vi "capstone2 ver 2.vi"() -> ()   [LabVIEW 2016]
uses:
  <instrlib>/Dynamixel Motor/Public/Motor Operation/Low Level/Baud Setting.ctl
  <vilib>/myRIO/Instrument Drivers/Onboard IO/DIO/typedefs/DIO Reference.ctl
  <vilib>/myRIO/Common/Instrument Driver Framework/Utilities/typedefs/myRIO Generic Hardware Reference.ctl
  <vilib>/myRIO/Common/Instrument Driver Framework/Utilities/typedefs/Hardware Version Enum.ctl
  <vilib>/myRIO/Common/Instrument Driver Framework/Utilities/typedefs/myRIO v1.0 Reference.ctl
  <vilib>/myRIO/Common/Instrument Driver Framework/Utilities/typedefs/Generic FPGA Reference.ctl
  <vilib>/myRIO/Common/Instrument Driver Framework/myRIO v1.0/DIO/typedefs/DIO Channels List.ctl
  <vilib>/myRIO/Common/Instrument Driver Framework/myRIO v1.0/DIO/typedefs/DIO Channels Enum.ctl
  <vilib>/userdefined/High Color/nirio_resource_hc.ctl
  <vilib>/myRIO/Common/Instrument Driver Framework/Utilities/vis/Is FPGA Ref Available.vi
  <vilib>/myRIO/Common/Instrument Driver Framework/myRIO v1.0/DIO/vis/myRIO v1.1 Open DIO.vi
  <vilib>/myRIO/Instrument Drivers/Onboard IO/DIO/vis/Write.vi
  <vilib>/myRIO/Common/Instrument Driver Framework/Utilities/vis/Validate Channels.vi
  <vilib>/myRIO/Common/Instrument Driver Framework/myRIO v1.0/DIO/vis/myRIO v1.0 Reserve DIO.vi
  <vilib>/myRIO/Common/Instrument Driver Framework/myRIO v1.0/UART/vis/myRIO v1.0 Close UART.vi
  <vilib>/myRIO/Common/Instrument Driver Framework/myRIO v1.0/Resource Manager/vis/myRIO v1.0 Reserve Channel List.vi
  <vilib>/myRIO/Common/Instrument Driver Framework/myRIO v1.0/DIO/vis/myRIO v1.0 Build MUX Configuration DIO.vi
  <vilib>/myRIO/Common/Instrument Driver Framework/myRIO v1.0/Resource Manager/vis/myRIO v1.0 Reserve Channel.vi
  <vilib>/myRIO/Common/Instrument Driver Framework/myRIO v1.0/Resource Manager/vis/myRIO v1.0 Unreserve Channel.vi
  <vilib>/myRIO/Common/Instrument Driver Framework/myRIO v1.0/Resource Manager/vis/myRIO v1.0 Create Configuration List.vi
  <vilib>/myRIO/Common/Instrument Driver Framework/myRIO v1.0/Resource Manager/vis/myRIO v1.0 Build Mutex Name.vi
  <vilib>/Utility/VariantDataType/GetNumericInfo.vi
  <vilib>/Utility/error.llb/Error Cluster From Error Code.vi
  <vilib>/myRIO/Common/Instrument Driver Framework/myRIO v1.0/myRIO v1.1 Open.vi
  <vilib>/myRIO/Common/Instrument Driver Framework/Utilities/vis/IO Manager.vi
  <vilib>/myRIO/Common/Instrument Driver Framework/Utilities/vis/Configuration Manager.vi
  <vilib>/myRIO/Common/Instrument Driver Framework/myRIO v1.0/Resource Manager/vis/myRIO v1.0 Configure IO.vi
  <vilib>/myRIO/Common/Instrument Driver Framework/myRIO v1.0/myRIO v1.0 Close.vi
  <vilib>/myRIO/Common/Instrument Driver Framework/myRIO v1.0/DIO/vis/myRIO v1.0 Write DIO.vi
  <vilib>/myRIO/Common/Instrument Driver Framework/Utilities/vis/FPGA Ref Manager.vi
  <vilib>/myRIO/Common/Instrument Driver Framework/myRIO v1.0/myRIO v1.0 Reset FPGA.vi
  <vilib>/myRIO/Common/Instrument Driver Framework/myRIO v1.0/IRQ/vis/myRIO v1.0 IRQ Info FGV.vi
  <vilib>/myRIO/Common/Instrument Driver Framework/myRIO v1.0/IRQ/vis/myRIO v1.0 Timer IRQ Info FGV.vi
  <vilib>/myRIO/Common/Instrument Driver Framework/myRIO v1.0/IRQ/vis/myRIO v1.0 ISR Agent.vi
  <vilib>/myRIO/Express VI/Onboard Devices/LED/LED Express VI.xnode
  <vilib>/myRIO/Instrument Drivers/Onboard IO/DIO/vis/myRIO DIO Open.xnode
  <instrlib>/Dynamixel Motor/Dynamixel Motor.lvlib
  <vilib>/myRIO/Instrument Drivers/Onboard IO/DIO/DIO.lvlib
  <vilib>/myRIO/Instrument Drivers/Utilities/Utilities.lvlib
panel:
  in  "main stop":bool
  out "RT TCP Loop time":u32
  out "motor temp":cluster{"0":sgl, "1":sgl, "2":sgl, "3":sgl}
  out "value":T1
  out "TCP Read data":string
  in  "정지":bool
  out "error out":errorcluster
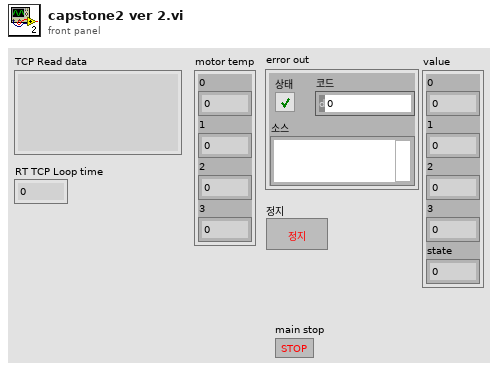
[diagram p1: front panel]
types:
  T1 = cluster{"0":sgl, "1":sgl, "2":sgl, "3":sgl, "state":sgl}
  T2 = typedef "DIO.lvlib/DIO Reference.ctl" = cluster{"myRIO Reference":T3, "DIO Channels List":T7}
  T3 = typedef "myRIO Generic Hardware Reference.ctl" = cluster{"myRIO Model":T4, "myRIO Hardware Reference":T5}
  T4 = typedef "Hardware Version Enum.ctl" = enum16{"Unknown", "myRIO-1900", "myRIO-1950", "roboRIO", "NI ELVIS RIO CM"}
  T5 = typedef "myRIO v1.0 Reference.ctl" = cluster{"Generic FPGA Reference":T6, "Allow multiple opens":bool}
  T6 = typedef "Generic FPGA Reference.ctl" = refnum<k20>
  T7 = typedef "DIO Channels List.ctl" = T8[]
  T8 = typedef "DIO Channels Enum.ctl" = enum16{"Not Connected", "C/DIO0", "C/DIO1", "C/DIO2", "C/DIO3", "C/DIO4", "C/DIO5", "C/DIO6", "C/DIO7", "A/DIO0", "A/DIO1", "A/DIO2", "A/DIO3", "A/DIO4", "A/DIO5", "A/DIO6", "A/DIO7", "A/DIO8", "A/DIO9", "A/DIO10", "A/DIO11", "A/DIO12", "A/DIO13", "A/DIO14", "A/DIO15", "B/DIO0", "B/DIO1", "B/DIO2", "B/DIO3", "B/DIO4", "B/DIO5", "B/DIO6", "B/DIO7", "B/DIO8", "B/DIO9", "B/DIO10", "B/DIO11", "B/DIO12", "B/DIO13", "B/DIO14", "B/DIO15", "LED0", "LED1", "LED2", "LED3", "Button0", "DIO/DIO0", "DIO/DIO1", "DIO/DIO2", "DIO/DIO3", "DIO/DIO4", "DIO/DIO5", "DIO/DIO6", "DIO/DIO7", "DIO/DIO8", "DIO/DIO9", "SPI/CS0", "SPI/CS1", "SPI/CS2", "SPI/CS3", "LED RADIO (Green)", "LED RADIO (Red)", "LED COMM (Green)", "LED COMM (Red)", "LED MODE (Green)", "LED MODE (Red)"}
  T9 = typedef "nirio_resource_hc.ctl" = tag
  T10 = cluster{"0":sgl, "1":sgl, "2":sgl, "3":sgl, "state":i32}
  T11 = typedef "Dynamixel Motor.lvlib/Baud Setting.ctl" = u8
  T12 = enum16{"big-endian, network order", "native, host order", "little-endian"}
  T13 = cluster{"Temperature (C)":u8, "Temperature (C)":u8, "Temperature (C)":u8, "Temperature (C)":u8}
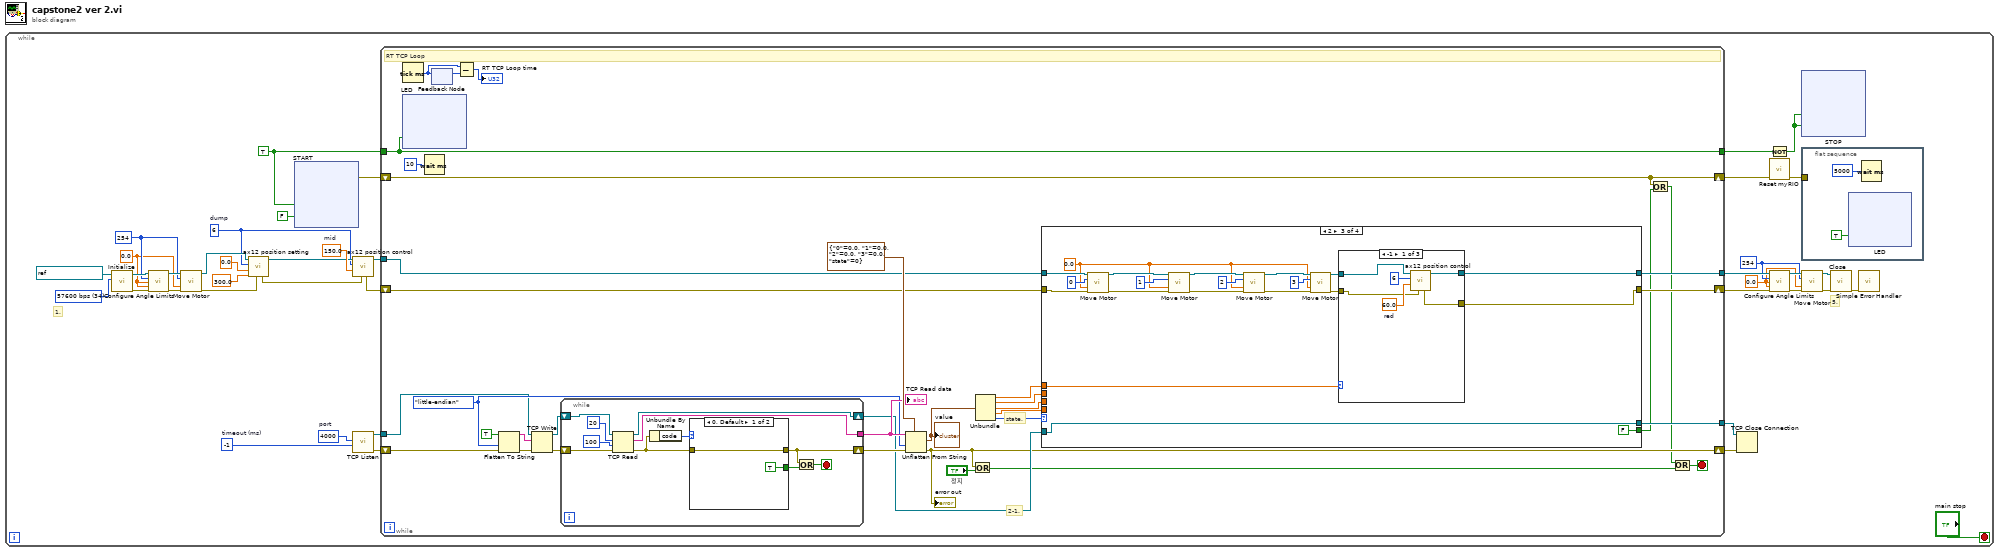
[diagram p0: block diagram]
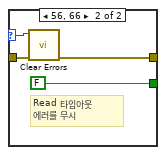
[diagram p2: hidden frame]
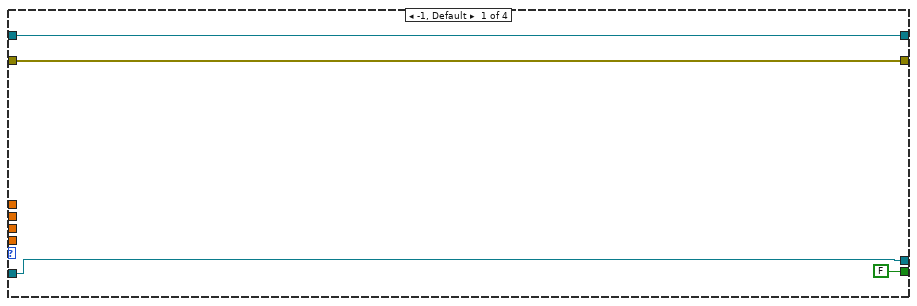
[diagram p3: hidden frame]
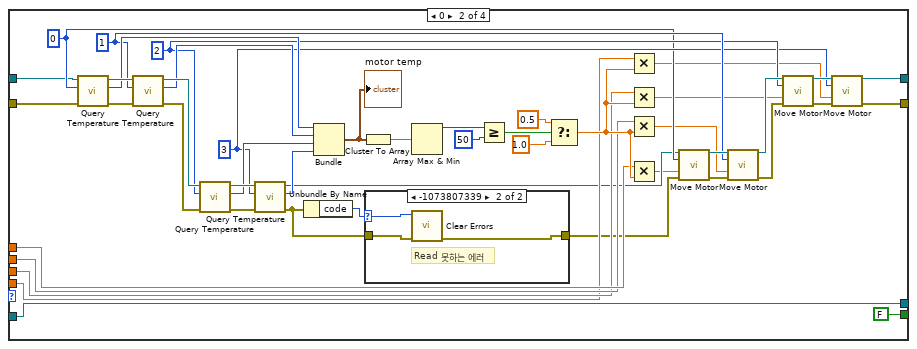
[diagram p4: hidden frame]
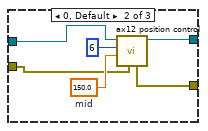
[diagram p6: hidden frame]
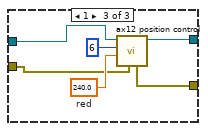
[diagram p7: hidden frame]
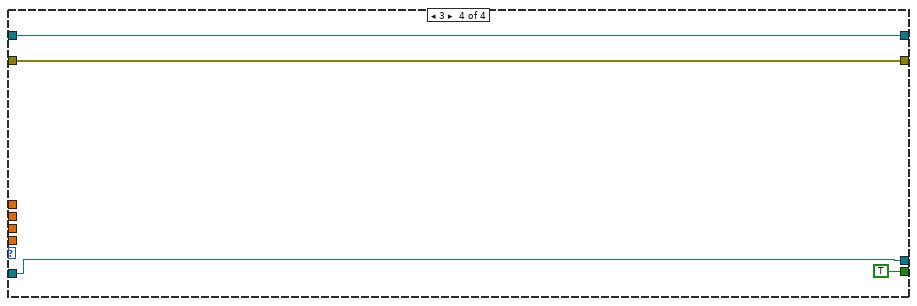
[diagram p8: hidden frame]
diagram:
  n1 = while {
    stop <- "main stop" stop-if-true
    w6 = 150.0  # mid
    w4 = 6  # dump
    w36 = T11 34 items=["1,000,000 bps"=1, "500,000 bps"=3, "400,000 bps"=4, "250,000 bps"=7, "200,000 bps"=9, "115200 bps"=16, "57600 bps"=34, "19200 bps"=103, "9600 bps"=207] ("Baud rate (57600 bps)")
    w26 = TRUE
    w16 = 0.0 ("Goal Speed (RPM)")
    w17 = u8 254 ("Motor ID (0)")
    w28 = u8 254 ("Motor ID (0)")
    w27 = 0.0 ("Clockwise Angle Limit (0 deg)")
    w40 = u16 4000  # port
    w41 = -1  # timeout (ms)
    # "5."
    # "1."
    n2 = call <instrlib>:"Initialize.vi"("Baud rate (57600 bps)"=w36, "VISA resource name"=refnum<visa-resource-name> "ASRL3::INSTR") -> ("error out"=w32:errorcluster, "VISA resource name out"=w31:refnum<visa-resource-name>)  [unwired: 8 in]
    n3 = call <instrlib>:"Configure Angle Limits.vi"("VISA resource name"=w31, "Motor ID (0)"=w28, "Clockwise Angle Limit (0 deg)"=w27, "Counter-Clockwise Angle Limit (300 deg)"=w27, "error in (no error)"=w32) -> ("VISA resource name out"=w30:refnum<visa-resource-name>, "error out"=w29:errorcluster)  [unwired: 9 in]
    n4 = call <instrlib>:"Move Motor.vi"("VISA resource name"=w30, "Motor ID (0)"=w28, "Goal Speed (RPM)"=w27, "error in (no error)"=w29) -> ("VISA resource name out"=w8:refnum<visa-resource-name>, "error out"=w7:errorcluster)  [unwired: 10 in]
    n5 = call "ax12 position setting.vi"("error in (no error)"=w7, "Counter-Clockwise Angle Limit (300 deg)"=300.0 ("Clockwise Angle Limit (0 deg)"), "Clockwise Angle Limit (0 deg)"=0.0, "Motor ID (0)"=w4, "VISA resource name"=w8) -> ("VISA resource name out"=w5:refnum<visa-resource-name>, "error out"=w1:errorcluster)  [unwired: 5 in]
    n6 = xnode "START"("LED0"=w26, "LED3"=FALSE) -> ("error out"=w12:errorcluster)  [unwired: 1 in]
    n7 = call "ax12 position control.vi"("error in (no error)"=w1, "Goal Position (180 deg)"=w6, "Motor ID (0)"=w4, "VISA resource name"=w5) -> ("VISA resource name out"=w3:refnum<visa-resource-name>, "error out"=w2:errorcluster)  [unwired: 6 in]
    n8 = call <vilib>:"TCP Listen.vi"("timeout ms (wait forever: -1)"=w41, "port"=w40) -> ("error out"=w37:errorcluster, "connection ID"=w23:refnum<k5>)  [unwired: 5 in, 3 out]
    n9 = while {
      tunnel: w23 -> [w161]
      tunnel: [w166] -> w39
      shift-right: [w157] -> w38
      shift-left: w37 -> [w158]
      shift-right: [w173] -> w21
      shift-left: w2 -> [w172]
      tunnel: w26 -> [w181]
      tunnel: [w181] -> w34
      tunnel: [w174] -> w19
      shift-right: [w152] -> w11
      shift-left: w12 -> [w152]
      tunnel: w3 -> [w154]
      stop <- w155 stop-if-true
      w162 = T12."little-endian" ("byte order (0:big-endian, network order)")
      # "state."
      # "2-1."
      # "RT TCP Loop"
      n10 = Tick Count (ms)() -> (millisecond timer value=w170:u32)
      n11 = xnode "LED"("LED1"=w181) -> ()  [unwired: 1 in, 1 out]
      n12 = Wait (ms)(milliseconds to wait=u32 10 ("대기 시간 (ms)")) -> ()  [unwired: 1 out]
      n13 = feedback #1() -> (w171:u32)  [unwired: 1 in]
      n14 = feedback-in #1(w170) -> ()
      n15 = Subtract(x=w170, y=w171) -> (x-y=→"RT TCP Loop time":u32)
      n16 = Flatten To String(anything=TRUE, byte order (0:big-endian, network order)=w162, error in (no error)=w158) -> (data string=w165:string, error out=w164:errorcluster)  [unwired: 1 in, 1 out]
      n17 = TCP Write(connection ID=w161, data in=w165, error in (no error)=w164) -> (connection ID out=w160:refnum<k5>, error out=w159:errorcluster)  [unwired: 1 in, 1 out]
      n18 = while {
        tunnel: [w194] -> w183
        shift-right: [w193] -> w167
        shift-left: w160 -> [w192]
        shift-right: [w188] -> w182
        shift-left: w159 -> [w191]
        stop <- w186 stop-if-true
        n19 = TCP Read(connection ID=w192, bytes to read=20 ("읽을 바이트"), error in (no error)=w191, 9:100 ("타임아웃 ms (25000)")) -> (connection ID out=w193:refnum<k5>, data out=w194:string, error out=w189:errorcluster)  [unwired: 1 in]
        n20 = Unbundle By Name(w189) -> ("code"=w190:i32)
        n21 = case shown="0, Default" w190 {
          selector: w190 -> [_ w201]
          tunnel: [w198 w200] -> w188
          tunnel: w189 -> [w198 w202]
          tunnel: [TRUE FALSE] -> w187
          frame 0, Default {
          }
          frame 56, 66 {
            # "Read 타임아웃\n에러를 무시"
            n22 = call <vilib>:"Clear Errors.vi"("error in (no error)"=w202, "specific error code to clear (0: all)"=w201) -> ("error out"=w200:errorcluster)  [unwired: 4 in, 1 out]
          }
        }
        n23 = Or(x=w188, y=w187) -> (x .or. y?=w186:bool)
      }
      "TCP Read data" <- w183
      n24 = Unflatten From String(type=T10 {"0"=0.0, "1"=0.0, "2"=0.0, "3"=0.0, "state"=0}, binary string=w183, byte order (0:big-endian, network order)=w162, error in (no error)=w182) -> (value=w180:T10, error out=w157:errorcluster)  [unwired: 1 in, 1 out]
      "error out" <- w157
      "value" <- w180
      n25 = Or(x=w157, y="정지") -> (x .or. y?=w151:bool)
      n26 = Unbundle(w180) -> ("0"=w179:sgl, "1"=w177:sgl, "2"=w178:sgl, "3"=w176:sgl, "state"=w175:i32)
      n27 = case shown="2" w175 {
        tunnel: w179 -> [_ w236 w263 _]
        tunnel: w177 -> [_ w235 _ _]
        tunnel: w178 -> [_ w234 _ _]
        tunnel: w176 -> [_ w233 _ _]
        tunnel: [w206 w218 w260 w295] -> w174
        tunnel: [w205 w219 w259 w296] -> w173
        tunnel: w172 -> [w205 w216 w273 w296]
        tunnel: w154 -> [w206 w209 w272 w295]
        tunnel: w167 -> [w204 w208 w258 w298]
        tunnel: [w204 w208 w258 w298] -> w166
        tunnel: [FALSE FALSE FALSE TRUE] -> w153
        frame -1, Default {
        }
        frame 0 {
          w220 = 3
          w221 = 2
          w222 = 1
          w217 = 0
          n28 = call <instrlib>:"Query Temperature.vi"("error in"=w216, "Motor ID (0)"=w217, "VISA resource name"=w209) -> ("error out"=w243:errorcluster, "Temperature (C)"=w232:u8, "VISA resource name out"=w246:refnum<visa-resource-name>)  [unwired: 6 in]
          n29 = call <instrlib>:"Query Temperature.vi"("error in"=w243, "Motor ID (0)"=w222, "VISA resource name"=w246) -> ("error out"=w242:errorcluster, "Temperature (C)"=w231:u8, "VISA resource name out"=w245:refnum<visa-resource-name>)  [unwired: 6 in]
          n30 = call <instrlib>:"Query Temperature.vi"("error in"=w242, "Motor ID (0)"=w221, "VISA resource name"=w245) -> ("error out"=w241:errorcluster, "Temperature (C)"=w230:u8, "VISA resource name out"=w244:refnum<visa-resource-name>)  [unwired: 6 in]
          n31 = call <instrlib>:"Query Temperature.vi"("error in"=w241, "Motor ID (0)"=w220, "VISA resource name"=w244) -> ("error out"=w223:errorcluster, "Temperature (C)"=w229:u8, "VISA resource name out"=w215:refnum<visa-resource-name>)  [unwired: 6 in]
          n32 = Unbundle By Name(w223) -> ("code"=w224:i32)
          n33 = Bundle("Temperature (C)"=w232, "Temperature (C)"=w231, "Temperature (C)"=w230, "Temperature (C)"=w229) -> (w226:T13)  [unwired: 1 in]
          "motor temp" <- w226
          n34 = Cluster To Array(cluster=w226) -> (array=w228:u8[])
          n35 = case shown="-1073807339" w224 {
            selector: w224 -> [_ w255]
            tunnel: [w253 w254] -> w214
            tunnel: w223 -> [w253 w256]
            frame 0, Default {
            }
            frame -1073807339 {
              # "Read 못하는 에러"
              n36 = call <vilib>:"Clear Errors.vi"("error in (no error)"=w256, "specific error code to clear (0: all)"=w255) -> ("error out"=w254:errorcluster)  [unwired: 4 in, 1 out]
            }
          }
          n37 = Array Max & Min(array=w228) -> (max value=w227:u8)  [unwired: 3 out]
          n38 = Greater Or Equal?(x=w227, y=50) -> (x >= y?=w225:bool)
          n39 = Select(t=0.5, s=w225, f=1.0) -> (s? t:f=w237:dbl)
          n40 = Multiply(x=w233, y=w237) -> (x*y=w210:dbl)
          n41 = Multiply(x=w234, y=w237) -> (x*y=w211:dbl)
          n42 = Multiply(x=w235, y=w237) -> (x*y=w212:dbl)
          n43 = Multiply(x=w236, y=w237) -> (x*y=w213:dbl)
          n44 = call <instrlib>:"Move Motor.vi"("VISA resource name"=w215, "Motor ID (0)"=w217, "Goal Speed (RPM)"=w213, "error in (no error)"=w214) -> ("VISA resource name out"=w247:refnum<visa-resource-name>, "error out"=w248:errorcluster)  [unwired: 10 in]
          n45 = call <instrlib>:"Move Motor.vi"("VISA resource name"=w247, "Motor ID (0)"=w222, "Goal Speed (RPM)"=w212, "error in (no error)"=w248) -> ("VISA resource name out"=w249:refnum<visa-resource-name>, "error out"=w251:errorcluster)  [unwired: 10 in]
          n46 = call <instrlib>:"Move Motor.vi"("VISA resource name"=w249, "Motor ID (0)"=w221, "Goal Speed (RPM)"=w211, "error in (no error)"=w251) -> ("VISA resource name out"=w250:refnum<visa-resource-name>, "error out"=w252:errorcluster)  [unwired: 10 in]
          n47 = call <instrlib>:"Move Motor.vi"("VISA resource name"=w250, "Motor ID (0)"=w220, "Goal Speed (RPM)"=w210, "error in (no error)"=w252) -> ("VISA resource name out"=w218:refnum<visa-resource-name>, "error out"=w219:errorcluster)  [unwired: 10 in]
        }
        frame 2 {
          w264 = 0.0 ("Goal Speed (RPM)")
          n48 = call <instrlib>:"Move Motor.vi"("VISA resource name"=w272, "Motor ID (0)"=u8 0, "Goal Speed (RPM)"=w264, "error in (no error)"=w273) -> ("VISA resource name out"=w271:refnum<visa-resource-name>, "error out"=w276:errorcluster)  [unwired: 10 in]
          n49 = call <instrlib>:"Move Motor.vi"("VISA resource name"=w271, "Motor ID (0)"=u8 1, "Goal Speed (RPM)"=w264, "error in (no error)"=w276) -> ("VISA resource name out"=w270:refnum<visa-resource-name>, "error out"=w275:errorcluster)  [unwired: 10 in]
          n50 = call <instrlib>:"Move Motor.vi"("VISA resource name"=w270, "Motor ID (0)"=u8 2, "Goal Speed (RPM)"=w264, "error in (no error)"=w275) -> ("VISA resource name out"=w269:refnum<visa-resource-name>, "error out"=w274:errorcluster)  [unwired: 10 in]
          n51 = call <instrlib>:"Move Motor.vi"("VISA resource name"=w269, "Motor ID (0)"=u8 3, "Goal Speed (RPM)"=w264, "error in (no error)"=w274) -> ("VISA resource name out"=w262:refnum<visa-resource-name>, "error out"=w261:errorcluster)  [unwired: 10 in]
          n52 = case shown="-1" w263 {
            tunnel: w262 -> [w281 w287 w293]
            tunnel: w261 -> [w280 w286 w292]
            tunnel: [w279 w284 w290] -> w260
            tunnel: [w278 w285 w291] -> w259
            frame -1 {
              w282 = 60.0  # red
              n53 = call "ax12 position control.vi"("error in (no error)"=w280, "Goal Position (180 deg)"=w282, "Motor ID (0)"=u8 6, "VISA resource name"=w281) -> ("VISA resource name out"=w279:refnum<visa-resource-name>, "error out"=w278:errorcluster)  [unwired: 6 in]
            }
            frame 0, Default {
              w288 = 150.0  # mid
              n54 = call "ax12 position control.vi"("error in (no error)"=w286, "Goal Position (180 deg)"=w288, "Motor ID (0)"=u8 6, "VISA resource name"=w287) -> ("VISA resource name out"=w284:refnum<visa-resource-name>, "error out"=w285:errorcluster)  [unwired: 6 in]
            }
            frame 1 {
              w294 = 240.0  # red
              n55 = call "ax12 position control.vi"("error in (no error)"=w292, "Goal Position (180 deg)"=w294, "Motor ID (0)"=u8 6, "VISA resource name"=w293) -> ("VISA resource name out"=w290:refnum<visa-resource-name>, "error out"=w291:errorcluster)  [unwired: 6 in]
            }
          }
        }
        frame 3 {
        }
      }
      n56 = Or(x=w152, y=w153) -> (x .or. y?=w156:bool)
      n57 = Or(x=w156, y=w151) -> (x .or. y?=w155:bool)
    }
    n58 = TCP Close Connection(connection ID=w39, error in (no error)=w38) -> ()  [unwired: 3 out]
    n59 = Not(x=w34) -> (.not. x?=w33:bool)
    n60 = call <vilib>:"Reset myRIO.vi"("error in (no error)"=w11) -> ("error out"=w15:errorcluster)  [unwired: 10 in]
    n61 = call <instrlib>:"Configure Angle Limits.vi"("VISA resource name"=w19, "Motor ID (0)"=w17, "Clockwise Angle Limit (0 deg)"=w16, "Counter-Clockwise Angle Limit (300 deg)"=w16, "error in (no error)"=w21) -> ("VISA resource name out"=w18:refnum<visa-resource-name>, "error out"=w20:errorcluster)  [unwired: 9 in]
    n62 = xnode "STOP"("LED0"=w33, "LED1"=w33) -> ()  [unwired: 1 in, 1 out]
    n63 = flat-sequence {
      tunnel: w15 -> [_]
      frame #0 {
        n64 = xnode "LED"("LED3"=TRUE) -> ()  [unwired: 1 in, 1 out]
        n65 = Wait (ms)(milliseconds to wait=5000) -> ()  [unwired: 1 out]
      }
    }
    n66 = call <instrlib>:"Move Motor.vi"("VISA resource name"=w18, "Motor ID (0)"=w17, "Goal Speed (RPM)"=w16, "error in (no error)"=w20) -> ("VISA resource name out"=w25:refnum<visa-resource-name>, "error out"=w24:errorcluster)  [unwired: 10 in]
    n67 = call <instrlib>:"Close.vi"("error in (no error)"=w24, "VISA resource name"=w25) -> ("error out"=w22:errorcluster)  [unwired: 9 in]
    n68 = call <vilib>:"Simple Error Handler.vi"("error in (no error)"=w22) -> ()  [unwired: 4 in, 5 out]
  }
